vi "Handle Error -8999-8997.vi"(8 "Tx Error":errorcluster, 11 "Message Enqueuer in":refnum<class "Message Enqueuer.lvclass">) -> (0 "Error Out":errorcluster)   [LabVIEW 2015, in "CS++LNA.lvlib"]
doc: "Send CS++LNAMessage object with error info to Message Enqueuer (typically enqueuer of neseted LNA).\n\nHandle error code -8999 -8997 set in CS++LNAMessage.lvclass:Do.vi\nMessage class from RLNA not found or bad typecast, empty or malformed. (Receiver)"
uses:
  CS++LNA.lvlib
  <vilib>/NI/Actors/Linked Network Actor/Linked Network Actor Messages/Transmit Network Message Msg/Transmit Network Message Msg.lvclass
  CS++LNAMessage/CS++LNAMessage.lvclass
  <vilib>/ActorFramework/Message Enqueuer/Message Enqueuer.lvclass
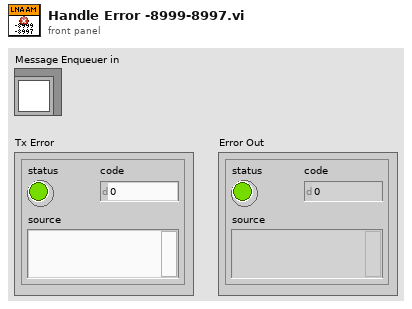
[diagram p1: front panel]
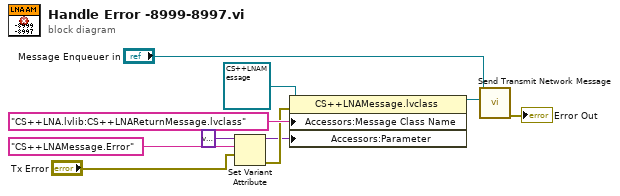
[diagram p0: block diagram]
diagram:
  n1 = Set Variant Attribute(Variant=variant, name="CS++LNAMessage.Error", value="Tx Error") -> (Variant out=w6:variant, error out=w9:errorcluster)  [unwired: 1 in, 1 out]
  n2 = property class="CS++LNAMessage.lvclass"(reference=refnum<class "CS++LNAMessage.lvclass"> refnum ("CS++LNA.lvlib:CS++LNAMessage.lvclass"), error in=w9, "Accessors:Message Class Name"="CS++LNA.lvlib:CS++LNAReturnMessage.lvclass" ("Message Class Name"), "Accessors:Parameter"=w6) -> (reference out=w4:refnum<class "CS++LNAMessage.lvclass">)  [unwired: 1 out]
  n3 = call <vilib>:"Send Transmit Network Message.vi"("Message"=w4, "Message Enqueuer"="Message Enqueuer in") -> ("error out"=→"Error Out":errorcluster)  [unwired: 8 in, 1 out]
